vi "PYTHON Execute Script__ogtk.vi"(4 "error in (no error)":errorcluster, 7 "Python Session in":T1) -> (0 "error out":errorcluster, 3 "Python Session out":T1)   [LabVIEW 2014]
doc: "This function compiles the previously assigned script text, if this hasn't already be done and then evaluates the compiled script. Before calling this you should have assigned all necessary input variables to this session, as they are required during evalution of the compiled script.\nThis function can be called multiple times for the same script with new assignments to only the input variables which have changed and the compiled script will then each time be reevaluated."
uses:
  <userlib>/_OpenG.lib/labpython/labpython.llb/PYTHON Session Refnum__ogtk.ctl
  <userlib>/_OpenG.lib/labpython/lvpython.dll
panel:
  # "PYTHON Execute Script.vi\n\nCompile and evaluate the script in the session context\n\nCopyright (C) 2002 Rolf Kalbermatter rolf.kalbermatter@citeng.com\nCopyright (C) 2002 James Kring jim@jimkring.com\n\nPlease visit http://www.OpenG.org to learn about the\nOpen Source LabVIEW software movement.\n\nThis library is free software; you can redistribute it and/or\nmodify it under the terms of the GNU Lesser General Public\nLicense as published by the Free Software Foundation; either\nversion 2.1 of the License, or (at your option) any later version.\nThis library is distributed in the hope that it will be useful,\nbut WITHOUT ANY WARRANTY; without even the implied warranty of\nMERCHANTABILITY or FITNESS FOR A PARTICULAR PURPOSE. See the GNU\nLesser General Public License for more details.\nYou should have received a copy of the GNU Lesser General Public\nLicense along with this library; if not, write to the Free Software\nFoundation, Inc., 59 Temple Place, Suite 330, Boston, MA 02111-1307 USA"
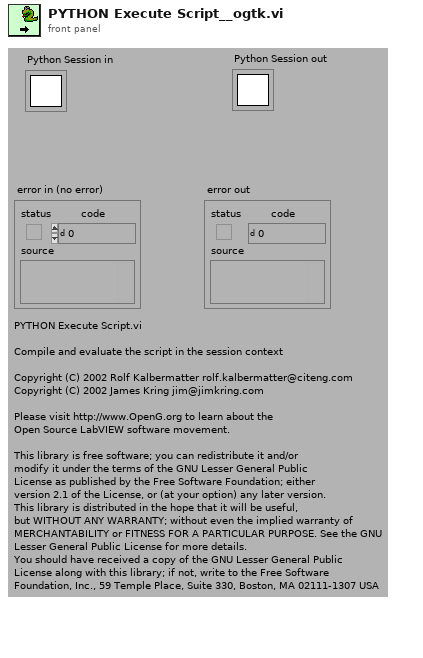
[diagram p1: front panel]
types:
  T1 = typedef "PYTHON Session Refnum__ogtk.ctl" = refnum<k1>
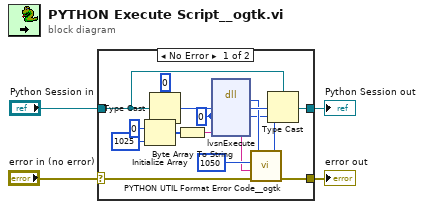
[diagram p0: block diagram]
diagram:
  n1 = case shown="No Error" "error in (no error)" {
    selector: "error in (no error)" -> [w14 w22]
    tunnel: [w8 w21] -> w1
    tunnel: [w12 w22] -> w3
    tunnel: "Python Session in" -> [w7 w21]
    frame No Error {
      w19 = 0 ("errStart")
      n2 = Initialize Array(u8 0 ("Element Data"), 1025 ("Dimension Size")) -> (w16:u8[])
      n3 = Type Cast(type=u32 0 ("session"), x=w7) -> (*(type *) &x=w9:u32)
      n4 = Byte Array To String(unsigned byte array=w16) -> (string=w15:string)
      n5 = dll-call lib="C:/Program Files (x86)/National Instruments/LabVIEW 2014/user.lib/_OpenG.lib/labpython/lvpython.*" fn="lvsnExecute"("session"=w9, "errStart"=w19, "errEnd"=w19, "errText"=w15) -> (w13:i32, "session"=w20:u32, "errStart"=w5:i32, "errText"=w6:string)  [unwired: 4 in, 2 out]
      n6 = call <userlib>:"PYTHON UTIL Format Error Code__ogtk.vi"("lineno"=w5, "error in (no error)"=w14, "message"=w6, "code"=1050, "Bool32"=w13) -> ("error out"=w12:errorcluster)  [unwired: 2 in]
      n7 = Type Cast(type=w7, x=w20) -> (*(type *) &x=w8:T1)
    }
    frame Error {
    }
  }
  "error out" <- w3
  "Python Session out" <- w1
